vi "Process.vi"(8 "error in":errorcluster, 11 "Inst UI.Magneto":refnum<class "Inst UI.Magneto.lvclass">) -> (0 "error out":errorcluster, 3 "Inst UI.Magneto out":refnum<class "Inst UI.Magneto.lvclass">)   [LabVIEW 2019, in "Inst UI.Magneto.lvclass"]
doc: "---------------------------------------------------------------\nJKI State Machine Objects™\nhttp://jki.net/state-machine-objects/\nCopyright (C) 2005-2015, JKI <info@jki.net>\nALL RIGHTS RESERVEDJKI State Machine Objects (SMO) 1.0.0.5\nJKI - JKI\nCopyright (c) 2016, JKI"
uses:
  Inst UI.Magneto.lvclass
  C:/Program Files (x86)/National Instruments/LabVIEW 2019/vi.lib/JKI/JKI SMO/SMO/SMO.lvclass
  C:/Program Files (x86)/National Instruments/LabVIEW 2019/user.lib/LevyLab/Instrument Framework/SMOs/Instrument UI/Instrument UI.lvclass
  C:/Program Files (x86)/National Instruments/LabVIEW 2019/vi.lib/JKI/JKI SMO/SMO.UI/SMO.UI.lvclass
  Inst.Magneto/Typedefs/Inst.Magneto.Commands--Enum.ctl
  Inst.Magneto/Typedefs/Inst.Magneto.getAll--Cluster.ctl
  Inst.Magneto/Inst.Magneto.lvclass
  C:/Program Files (x86)/National Instruments/LabVIEW 2019/user.lib/LevyLab/Instrument Framework/SMOs/Instrument/Instrument.lvclass
  Inst UI.Magneto.UI--Cluster.ctl
  Inst.Magneto/Typedefs/Inst.Magneto.Configuration--Cluster.ctl
  <userlib>/LevyLab/Instrument Framework/SMOs/Configuration/Configuration.lvclass
  <userlib>/LevyLab/Instrument Framework/SMOs/RemoteControl/Typedefs/Message--Cluster.ctl
  <userlib>/LevyLab/Instrument Framework/SMOs/Instrument UI/Instrument UI.lvclass/Instrument UI.ctl
  Inst.Magneto/Inst.Magneto.lvclass/Inst.Magneto.ctl
  <vilib>/JKI/JKI SMO/SMO/SMO.lvclass/SMO.ctl
  <userlib>/LevyLab/Instrument Framework/SMOs/Configuration/Configuration.lvclass/Configuration.ctl
  <userlib>/LevyLab/Instrument Framework/SMOs/Instrument/Instrument.lvclass/Instrument.ctl
  <userlib>/LevyLab/Instrument Framework/SMOs/Instrument/Typedefs/Client Type--Enum.ctl
  36130e5c-4340-4b59-a0e3-69bc2d3aea66.vi
  09e9697b-516c-49fb-b2dc-692589121b6f.vi
  <vilib>/JKI/JKI SMO/SMO/Private/ReftoDVR--SMO.vi
  09e9697b-516c-49fb-b2dc-692589121b6f.vi/cc30aaa2-4cab-4253-82f5-7584654065fd.vi
  09e9697b-516c-49fb-b2dc-692589121b6f.vi/cc30aaa2-4cab-4253-82f5-7584654065fd.vi/c8a96f78-a4da-4a88-8425-6c4f2c11086a.vi
  <userlib>/LevyLab/Instrument Framework/SMOs/Instrument/API/Send and Receive.vi
  09e9697b-516c-49fb-b2dc-692589121b6f.vi/cc30aaa2-4cab-4253-82f5-7584654065fd.vi/d7be4ad8-201f-4865-b26c-b4f29c6f9adb.vi
  <userlib>/LevyLab/Instrument Framework/SMOs/Instrument/Private/Get Client Type.vi
  09e9697b-516c-49fb-b2dc-692589121b6f.vi/cc30aaa2-4cab-4253-82f5-7584654065fd.vi/c8a96f78-a4da-4a88-8425-6c4f2c11086a.vi/c8de3620-5771-48fc-a831-9cb6daefdad3.vi
  09e9697b-516c-49fb-b2dc-692589121b6f.vi/cc30aaa2-4cab-4253-82f5-7584654065fd.vi/c8a96f78-a4da-4a88-8425-6c4f2c11086a.vi/b35627d4-a654-4984-b331-4a3a395fed01.vi
  09e9697b-516c-49fb-b2dc-692589121b6f.vi/cc30aaa2-4cab-4253-82f5-7584654065fd.vi/d7be4ad8-201f-4865-b26c-b4f29c6f9adb.vi/f494a3ae-3c03-4931-987a-c87ab374a794.vi
  09e9697b-516c-49fb-b2dc-692589121b6f.vi/cc30aaa2-4cab-4253-82f5-7584654065fd.vi/d7be4ad8-201f-4865-b26c-b4f29c6f9adb.vi/582413b9-0fe2-481b-be04-b448e5fee34f.vi
  09e9697b-516c-49fb-b2dc-692589121b6f.vi/cc30aaa2-4cab-4253-82f5-7584654065fd.vi/d7be4ad8-201f-4865-b26c-b4f29c6f9adb.vi/f494a3ae-3c03-4931-987a-c87ab374a794.vi/0ff650d9-b68d-4108-b8b1-733b4d68d29e.vi
  09e9697b-516c-49fb-b2dc-692589121b6f.vi/cc30aaa2-4cab-4253-82f5-7584654065fd.vi/d7be4ad8-201f-4865-b26c-b4f29c6f9adb.vi/f494a3ae-3c03-4931-987a-c87ab374a794.vi/2f422144-46f9-473a-bbc2-4310a8f125b6.vi
  <vilib>/JDP Science/JSONtext/JSON text to Variant.vi
  <userlib>/LevyLab/Instrument Framework/SMOs/Instrument/Private/Get RC Connection Status.vi
  <userlib>/LevyLab/Instrument Framework/SMOs/RemoteControl/API/Send and Receive.vi
  <vilib>/Utility/Data Type/Get Type Information.vi
  <vilib>/JDP Science/JSONtext/Variant to JSON Text.vi
  <vilib>/National Instruments/GUID Generator/Guid Generator.vi
  <userlib>/LevyLab/Instrument Framework/SMOs/Instrument/Private/Instrument.MessageFromProcess.EventStructure.vi
  <userlib>/LevyLab/Instrument Framework/SMOs/Instrument/Instrument.lvclass
  <vilib>/JDP Science/JSONtext/LVClass Serializer/JSONtext LVClass Serializer.lvclass
  <userlib>/LevyLab/Instrument Framework/SMOs/Instrument UI/Instrument UI.lvclass
  <vilib>/JKI/JKI SMO/SMO/SMO.lvclass
  <vilib>/JKI/JKI SMO/SMO.UI/SMO.UI.lvclass
  <userlib>/LevyLab/Instrument Framework/SMOs/RemoteControl/RemoteControl.lvclass
panel:
  out "error out 2":errorcluster
  out "output array":dbl[][](array[numeric])
  out "B-field Values (sensor, x, y, z) uT":cluster{dbl[], dbl[], dbl[], dbl[]}
  out "coerced(x)":u32
  out "Sensor 0 B_y":dbl(graph)
  out "Sensor 0 B_x":dbl(graph)
  in  "STOP":bool
  # "SMO UI Template"
  # "For instructions on how to use the JKI State Machine Objects, examples and video tutorials, visit:\nhttp://jki.net/state-machine-objects/\n\nJKI State Machine Objects™\nhttp://jki.net/state-machine-objects/\nCopyright (C) 2005-2015, JKI <info@jki.net>\nALL RIGHTS RESERVED"
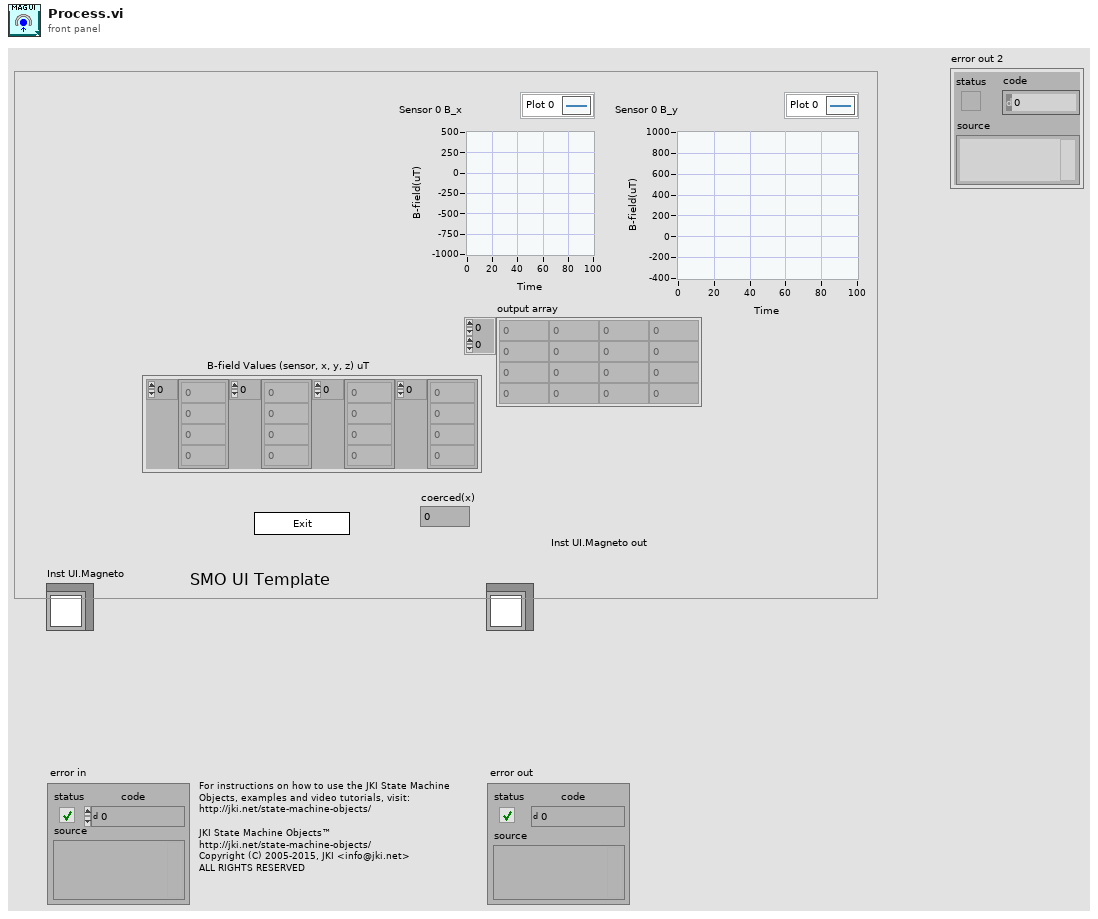
[diagram p1: front panel]
types:
  T1 = typedef "Inst.Magneto.lvclass/Inst.Magneto.Commands--Enum.ctl" = enum16{"GetRead", "Read", "Clear Values"}
  T2 = enum32{"invalid app kind", "Development System", "Run Time System", "Student Edition", "Embedded LabVIEW", "Evaluation", "Custom"}
  T3 = typedef "Inst.Magneto.lvclass/Inst.Magneto.getAll--Cluster.ctl" = cluster{"AllString":string}
  T4 = cluster{"Sensor":i32, "x":dbl, "y":dbl, "z":dbl}[]
  T5 = enum32{"Invalid", "Standard", "Closed", "Hidden", "Minimized", "Maximized"}
  T6 = typedef "Instrument.lvclass/Client Type--Enum.ctl" = enum16{"Remote", "Local"}
  T7 = typedef "Inst.Magneto.lvclass/Inst.Magneto.Configuration--Cluster.ctl" = cluster{"Server URL":string}
  T8 = typedef "Inst UI.Magneto.lvclass/Inst UI.Magneto.UI--Cluster.ctl" = cluster{"Parameter":dbl, "\nURL":string}
  T9 = typedef "RemoteControl.lvclass/Message--Cluster.ctl" = cluster{"Command":string, "Data":variant, "ID":string}
  T10 = cluster{"Core":cluster{"Current VI Reference":refnum<vi>, "Close Panel on Exit?":bool, "Last Error":cluster{"error":errorcluster, "previous state":string, "remaining states":string}, "Shutdown?":bool}, "Instrument UI":refnum<class "Inst UI.Magneto.lvclass">, "Instrument":refnum<class "Inst.Magneto.lvclass">, "Configuration":refnum<class "Configuration.lvclass">, "Config Cluster":T7, "getAll":T3, "UI Cluster":T8, "Message":T9}
  T11 = cluster{"Current VI Reference":refnum<vi>, "Close Panel on Exit?":bool, "Last Error":cluster{"error":errorcluster, "previous state":string, "remaining states":string}, "Shutdown?":bool}
  T12 = typedef "SMO.lvclass/Protected Events.ctl" = cluster{"StopProcesses":refnum<user-event>, "AbortProcesses":refnum<user-event>, "Config Changed":refnum<user-event>, "Dependency":refnum<user-event>}
  T13 = typedef "Instrument.lvclass/PublicEvents--Cluster.ctl" = cluster{"MessageFromProcess":refnum<user-event>}
  T14 = typedef "Inst.Magneto.lvclass/PublicEvents--Cluster.ctl" = cluster{"MessageFromProcess":refnum<user-event>}
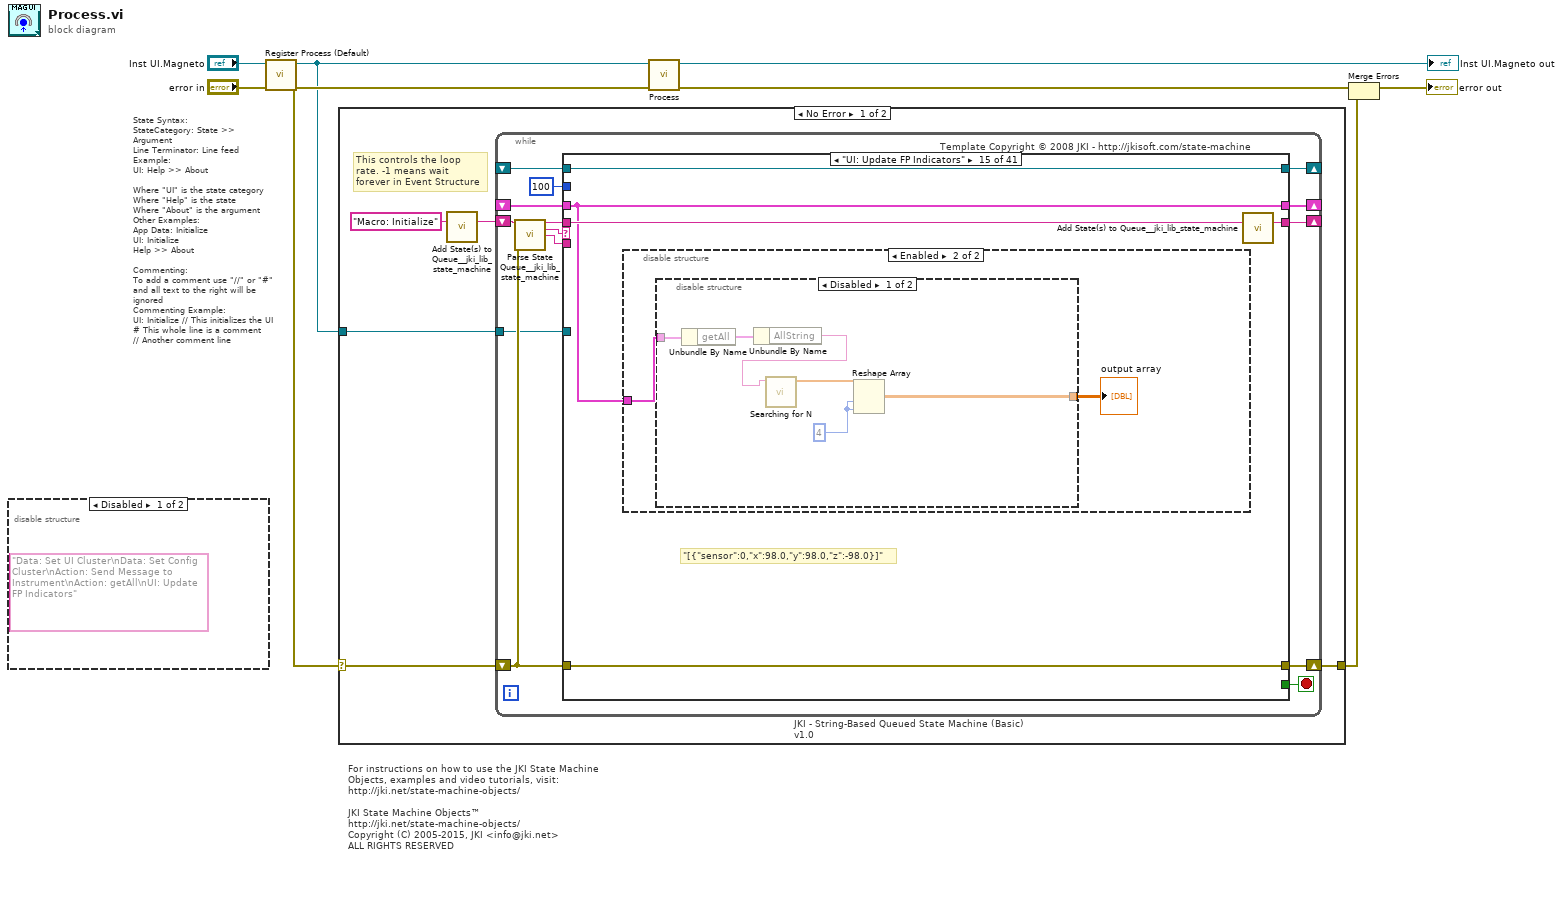
[diagram p0: block diagram]
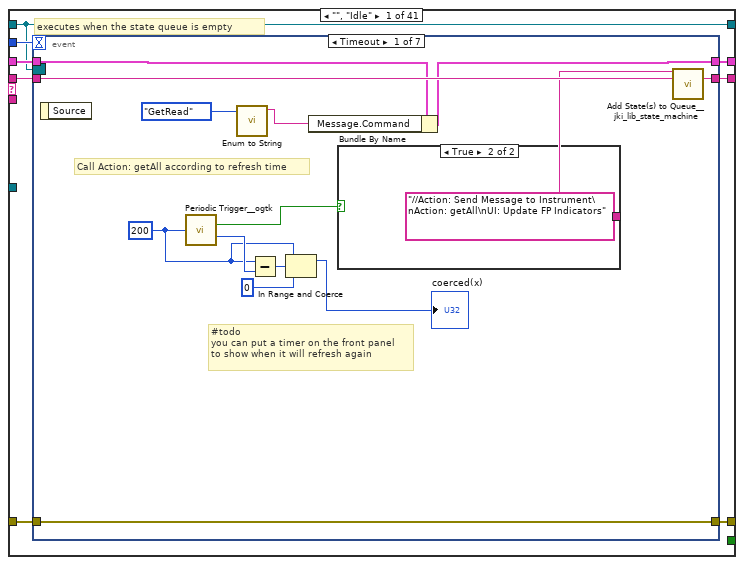
[diagram p3: hidden frame]
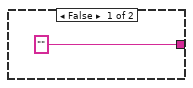
[diagram p4: hidden frame]
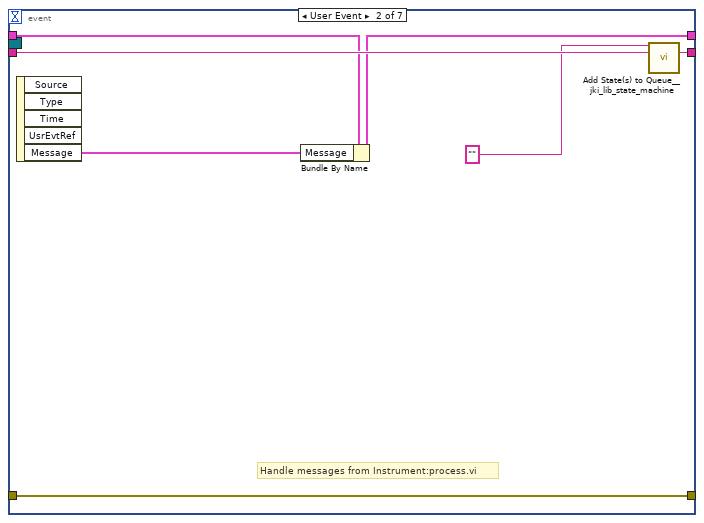
[diagram p5: hidden frame]
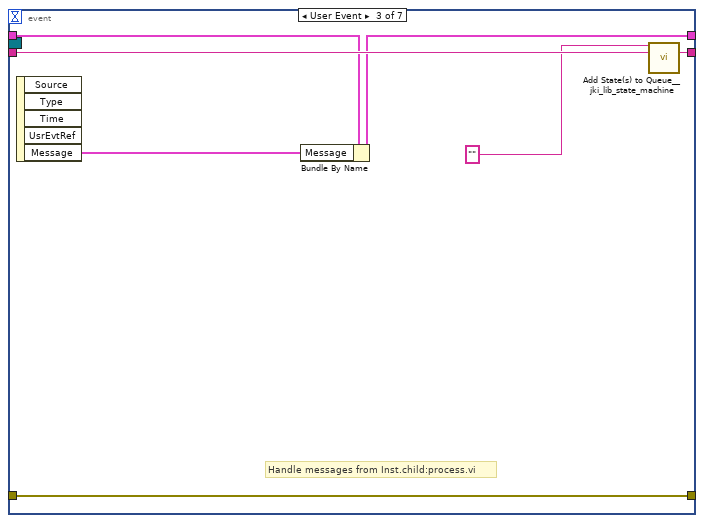
[diagram p6: hidden frame]
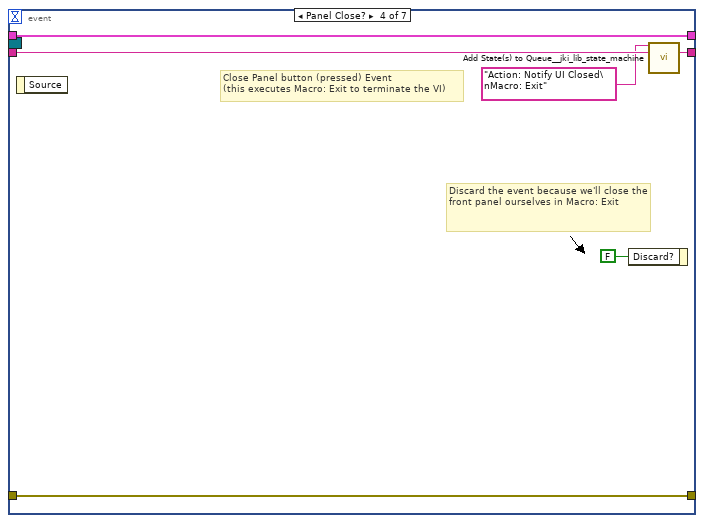
[diagram p7: hidden frame]
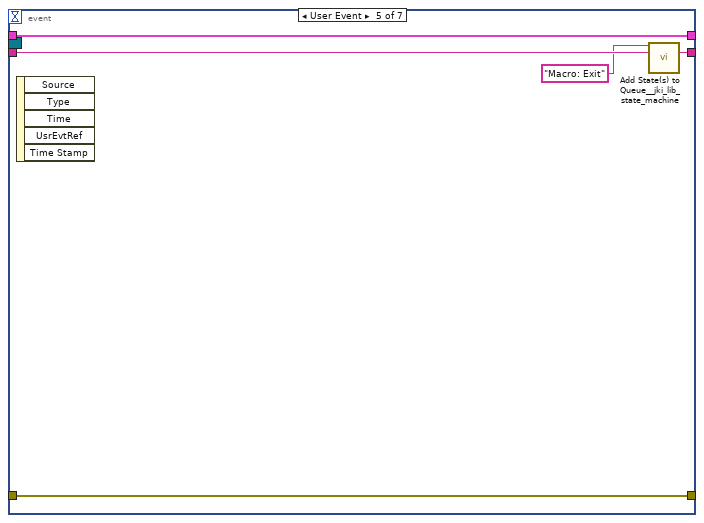
[diagram p8: hidden frame]
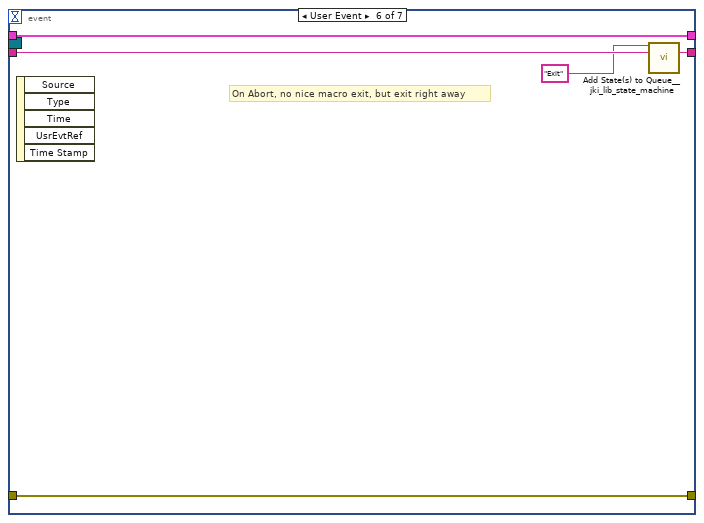
[diagram p9: hidden frame]
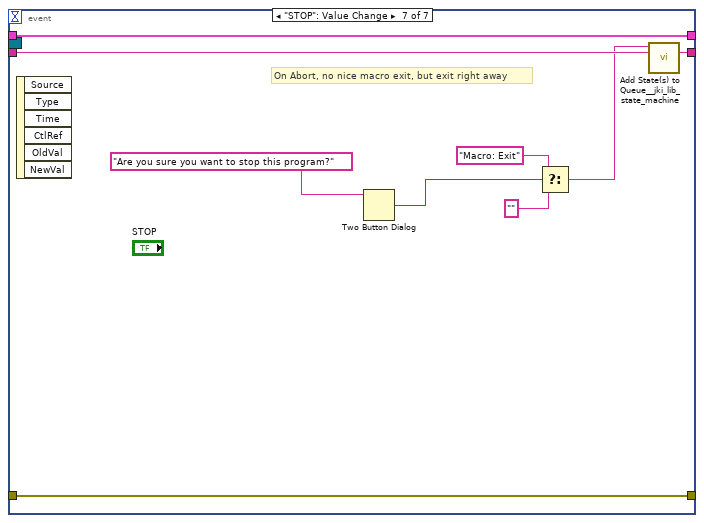
[diagram p10: hidden frame]
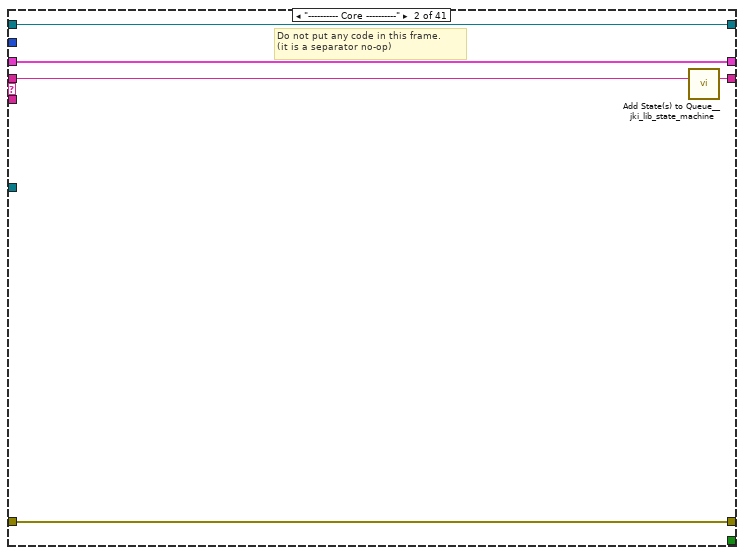
[diagram p11: hidden frame]
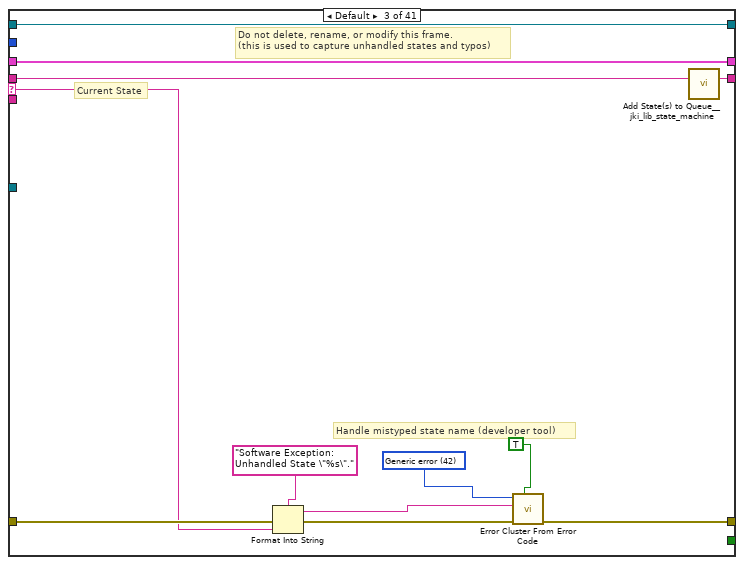
[diagram p12: hidden frame]
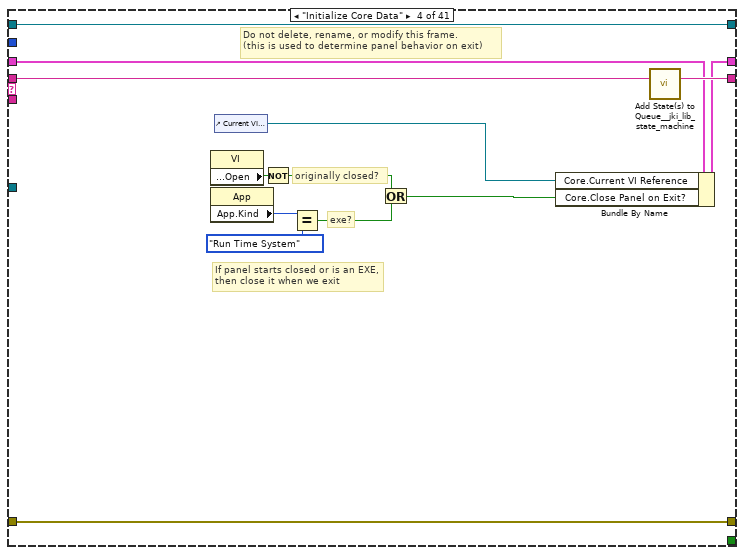
[diagram p13: hidden frame]
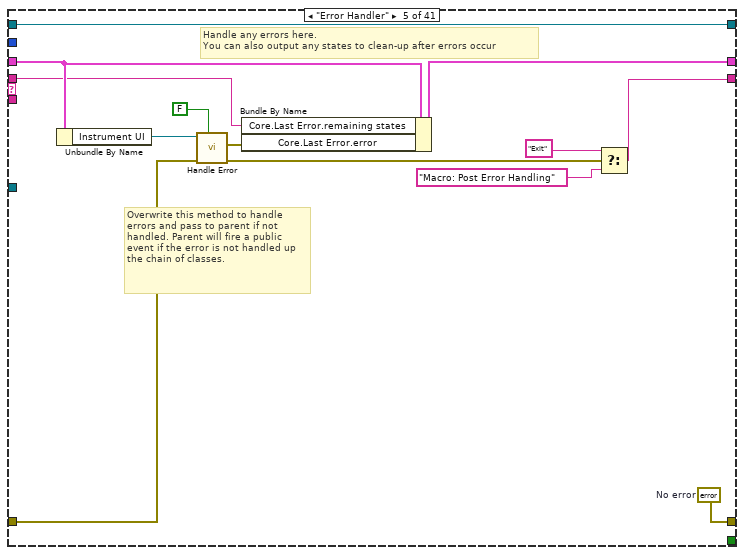
[diagram p14: hidden frame]
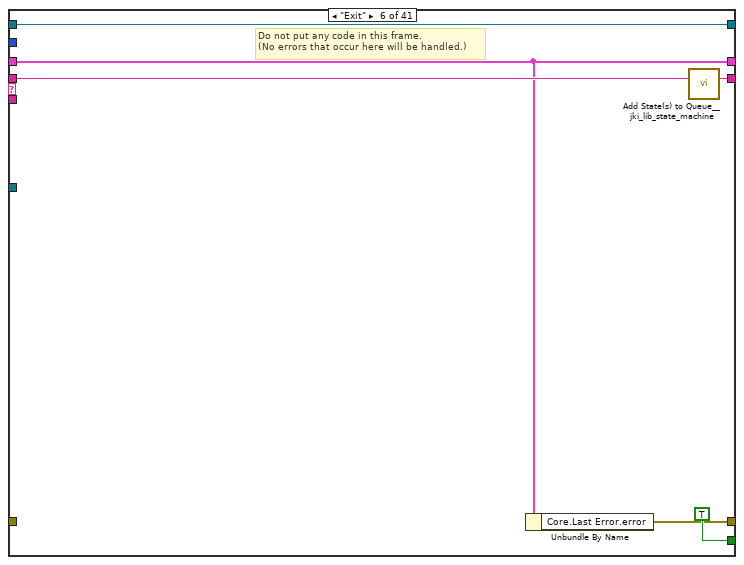
[diagram p15: hidden frame]
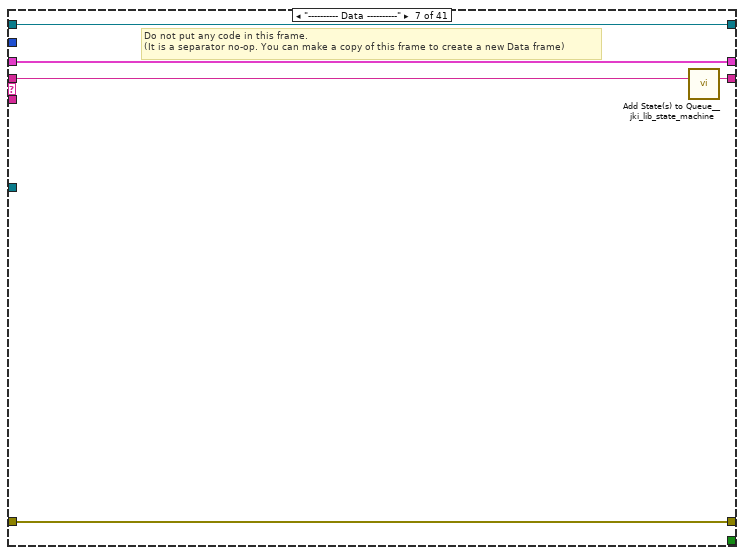
[diagram p16: hidden frame]
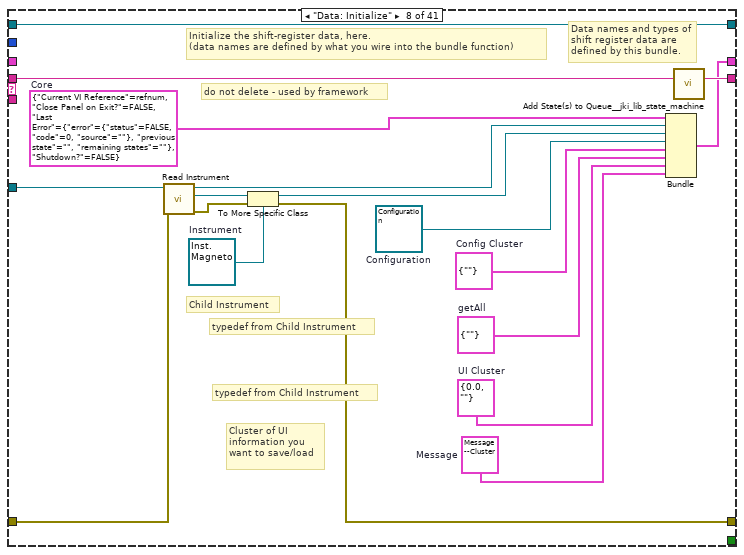
[diagram p17: hidden frame]
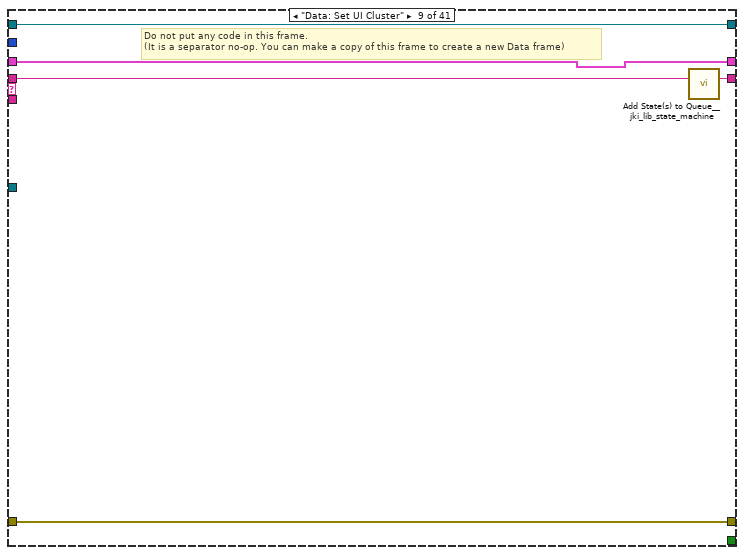
[diagram p18: hidden frame]
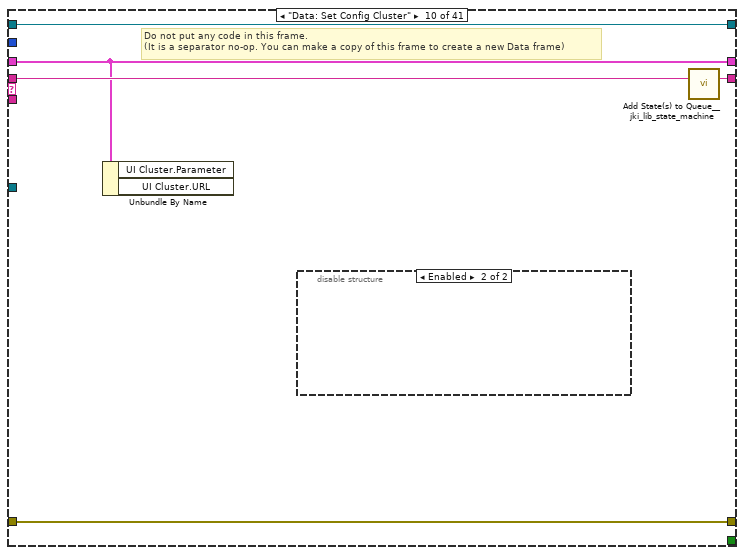
[diagram p19: hidden frame]
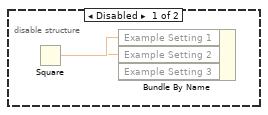
[diagram p20: hidden frame]
diagram:
  # "State Syntax:\nStateCategory: State >> Argument\nLine Terminator: Line feed\nExample:\nUI: Help >> About\n\nWhere \"UI\" is the state category\nWhere \"Help\" is the state\nWhere \"About\" is the argument\nOther Examples:\nApp Data: Initialize\nUI: Initialize\nHelp >> About\n\nCommenting:\nTo add a comment use \"//\" or \"#\" and all text to the right will be ignored\nCommenting Example:\nUI: Initialize // This initializes the UI\n# This whole line is a comment\n// Another comment line"
  # "For instructions on how to use the JKI State Machine Objects, examples and video tutorials, visit:\nhttp://jki.net/state-machine-objects/\n\nJKI State Machine Objects™\nhttp://jki.net/state-machine-objects/\nCopyright (C) 2005-2015, JKI <info@jki.net>\nALL RIGHTS RESERVED"
  n1 = disable-structure shown="Disabled" {
    frame Disabled {
      w9 = "Data: Set UI Cluster\nData: Set Config Cluster\nAction: Send Message to Instrument\nAction: getAll\nUI: Update FP Indicators" ("State(s) in Front (\"\")")
    }
    frame Enabled {
    }
  }
  n2 = call <vilib>:"Register Process (Default).vi"("error in (no error)"="error in", "SMO"="Inst UI.Magneto") -> ("error out"=w5:errorcluster, "SelfRef"=w4:refnum<class "Inst UI.Magneto.lvclass">)  [unwired: 8 in]
  n3 = case shown="No Error" w5 {
    selector: w5 -> [w11 w513]
    tunnel: w4 -> [w12 _]
    tunnel: [w10 w513] -> w1
    frame No Error {
      # "This controls the loop rate. -1 means wait forever in Event Structure"
      n4 = call <vilib>:"Add State(s) to Queue__jki_lib_state_machine.vi"("State(s) in (\"\")"="Macro: Initialize") -> ("States Out"=w14:string)  [unwired: 14 in]
      n5 = while "JKI - String-Based Queued State Machine (Basic) v1.0" {
        shift-right: [w21] -> _
        shift-left: _ -> [w20]
        shift-right: [w24] -> w10
        shift-left: w11 -> [w18]
        shift-right: [w23] -> _
        shift-left: w14 -> [w25]
        tunnel: w12 -> [w17]
        shift-right: [w16] -> _
        shift-left: _ -> [w15]
        stop <- w22 stop-if-true
        # "Template Copyright © 2008 JKI - http://jkisoft.com/state-machine"
        n6 = call <vilib>:"Parse State Queue__jki_lib_state_machine.vi"("State Queue"=w25, "Error In (no error)"=w18) -> ("Remaining States"=w27:string, "Current State"=w28:string, "Arguments"=w26:string)  [unwired: 11 in]
        n7 = case shown="\"UI: Update FP Indicators\"" w28 {
          selector: w28 -> [_ _ w98 _ _ _ _ _ _ _ _ _ _ _ _ _ _ _ _ _ _ _ _ _ _ _ _ _ _ _ _ _ _ _ _ _ _ _ _ _ _]
          tunnel: w27 -> [w36 w96 w102 w121 w125 w140 w145 w163 w168 w173 w183 w188 w195 w200 w205 w241 w257 w289 w298 w310 w320 w326 w341 w346 w357 w364 w369 w385 w391 w396 w411 w419 w431 w438 w445 w457 w470 w480 w491 w502 w512]
          tunnel: w26 -> [_ _ _ _ _ _ _ _ _ _ _ _ _ _ _ w235 w251 _ _ _ _ _ _ _ _ _ _ _ _ _ _ _ _ _ _ _ _ _ _ _ _]
          tunnel: w20 -> [w34 w93 w100 w112 w128 w136 w142 _ w164 w169 w177 w185 w193 w196 w201 w239 w253 w286 w294 w300 w317 w323 w328 w343 w354 w359 w366 w383 w389 w393 w404 w416 w422 w433 w439 w449 w464 w472 w486 w497 w507]
          tunnel: [w33 w94 w104 w118 w130 w135 w143 w150 w166 w171 w179 w186 w190 w198 w202 w236 w254 w287 w296 w308 w318 w324 w339 w344 w348 w360 w367 w380 w386 w394 w397 w414 w423 w435 w440 w454 w467 w477 w482 w493 w503] -> w24
          tunnel: w18 -> [w32 w94 w103 w118 w124 _ w143 w147 w166 w171 w180 w186 w191 w198 w202 w237 w255 w287 w296 w308 w318 w324 w339 w344 w349 w361 w367 w370 w387 w394 w406 w412 w424 w435 w441 w450 w459 w473 w483 w494 w504]
          tunnel: [w35 w95 w101 w120 w122 w139 w144 w162 w167 w172 w182 w187 w194 w199 w204 w240 w256 w288 w297 w309 w319 w325 w340 w345 w356 w363 w368 w384 w390 w395 w410 w418 w430 w437 w444 w456 w469 w479 w490 w501 w511] -> w23
          tunnel: [_ _ _ _ _ TRUE _ _ _ _ _ _ _ _ _ _ _ _ _ _ _ _ _ _ _ _ _ _ _ _ _ _ _ _ _ _ _ _ _ _ _] -> w22
          tunnel: [w31 w93 w100 w119 w127 w136 w142 w161 w164 w169 w177 w185 w193 w196 w201 w239 w253 w286 w294 w301 w317 w323 w328 w343 w354 w359 w366 w383 w389 w393 w408 w416 w420 w432 w439 w451 w465 w474 w487 w498 w508] -> w21
          tunnel: 100 ("Timeout") -> [w30 _ _ _ _ _ _ _ _ _ _ _ _ _ _ _ _ _ _ _ _ _ _ _ _ _ _ _ _ _ _ _ _ _ _ _ _ _ _ _ _]
          tunnel: w17 -> [_ _ _ _ _ _ _ w148 _ _ _ _ _ _ _ _ _ _ _ _ _ _ _ _ _ _ _ _ _ _ _ _ _ _ _ _ _ _ _ _ _]
          tunnel: [w29 w92 w97 w109 w134 w137 w141 w160 w165 w170 w178 w184 w192 w197 w203 w238 w250 w285 w295 w307 w316 w322 w333 w342 w355 w362 w365 w382 w388 w392 w409 w417 w429 w436 w443 w455 w468 w478 w489 w500 w510] -> w16
          tunnel: w15 -> [w29 w92 w97 w109 w134 w137 w141 w160 w165 w170 w178 w184 w192 w197 w203 w238 w250 w285 w295 w307 w316 w322 w333 w342 w355 w362 w365 _ w388 w392 w409 w417 w429 w436 w443 w455 w468 w478 w489 w500 w510]
          frame "", "Idle" {
            # "executes when the state queue is empty"
            n8 = event shown="[0] Timeout" {
              selector: w29 -> [_ _ _ _ _ _ _]
              dyn-events: _ -> [_ _ _ _ _ _ _]
              timeout: w30 -> [_ _ _ _ _ _ _]
              tunnel: w36 -> [w50 w59 w66 w72 w77 w82 w91]
              tunnel: [w49 w58 w65 w71 w76 w81 w90] -> w35
              tunnel: w34 -> [w39 w56 w63 w68 w74 w79 w88]
              tunnel: [w48 w57 w64 w67 w75 w80 w89] -> w33
              tunnel: w32 -> [w48 w57 w64 w67 w75 w80 w89]
              tunnel: [w40 w55 w62 w68 w74 w79 w88] -> w31
              event Timeout {
                w43 = u32 200 ("time (ms)")
                # "#todo\nyou can put a timer on the front panel\nto show when it will refresh again"
                # "Call Action: getAll according to refresh time"
                n9 = event-data() -> ()  [unwired: 1 in, 1 out]
                n10 = call <userlib>:"Periodic Trigger__ogtk.vi"("time (ms)"=w43) -> ("Triggered"=w47:bool, "timer value"=w46:u32)  [unwired: 12 in, 1 out]
                n11 = call <userlib>:"Enum to String.vi"("Command"=Inst.Magneto.Commands--Enum."GetRead" ("Commands")) -> ("Command"=w37:string)  [unwired: 9 in, 1 out]
                n12 = Subtract(x=w43, y=w46) -> (x-y=w45:u32)
                n13 = In Range and Coerce(upper limit=w43, x=w45, lower limit=u32 0) -> (coerced(x)=→"coerced(x)":u32)  [unwired: 1 out]
                n14 = Bundle By Name(cluster=w39, "Message.Command"=w37) -> (w40:T10)
                n15 = case shown="True" w47 {
                  tunnel: ["" ("State(s) in Front (\"\")") "//Action: Send Message to Instrument\nAction: getAll\nUI: Update FP Indicators" ("State(s) in Front (\"\")")] -> w41
                  frame False {
                  }
                  frame True {
                  }
                }
                n16 = call <vilib>:"Add State(s) to Queue__jki_lib_state_machine.vi"("State(s) in Front (\"\")"=w41, "State(s) in (\"\")"=w50) -> ("States Out"=w49:string)  [unwired: 13 in]
              }
              event User Event {
                # "Handle messages from Instrument:process.vi"
                n17 = event-data() -> ("Message"=w53:T9)  [unwired: 1 in, 4 out]
                n18 = Bundle By Name(cluster=w56, "Message"=w53) -> (w55:T10)
                n19 = call <vilib>:"Add State(s) to Queue__jki_lib_state_machine.vi"("State(s) in Front (\"\")"="" ("State(s) in Front (\"\")"), "State(s) in (\"\")"=w59) -> ("States Out"=w58:string)  [unwired: 13 in]
              }
              event User Event {
                # "Handle messages from Inst.child:process.vi"
                n20 = event-data() -> ("Message"=w60:T9)  [unwired: 1 in, 4 out]
                n21 = Bundle By Name(cluster=w63, "Message"=w60) -> (w62:T10)
                n22 = call <vilib>:"Add State(s) to Queue__jki_lib_state_machine.vi"("State(s) in Front (\"\")"="" ("State(s) in Front (\"\")"), "State(s) in (\"\")"=w66) -> ("States Out"=w65:string)  [unwired: 13 in]
              }
              event Panel Close? {
                # "Discard the event because we'll close the front panel ourselves in Macro: Exit"
                # "Close Panel button (pressed) Event\n(this executes Macro: Exit to terminate the VI)"
                n23 = event-data() -> ()  [unwired: 1 in, 1 out]
                n24 = event-data("Discard?"=FALSE) -> ()  [unwired: 1 in, 1 out]
                n25 = call <vilib>:"Add State(s) to Queue__jki_lib_state_machine.vi"("State(s) in Front (\"\")"="Action: Notify UI Closed\nMacro: Exit", "State(s) in (\"\")"=w72) -> ("States Out"=w71:string)  [unwired: 13 in]
              }
              event User Event {
                n26 = event-data() -> ()  [unwired: 1 in, 5 out]
                n27 = call <vilib>:"Add State(s) to Queue__jki_lib_state_machine.vi"("State(s) in Front (\"\")"="Macro: Exit", "State(s) in (\"\")"=w77) -> ("States Out"=w76:string)  [unwired: 13 in]
              }
              event User Event {
                # "On Abort, no nice macro exit, but exit right away"
                n28 = event-data() -> ()  [unwired: 1 in, 5 out]
                n29 = call <vilib>:"Add State(s) to Queue__jki_lib_state_machine.vi"("State(s) in Front (\"\")"="Exit", "State(s) in (\"\")"=w82) -> ("States Out"=w81:string)  [unwired: 13 in]
              }
              event "STOP": Value Change {
                # "On Abort, no nice macro exit, but exit right away"
                n30 = event-data() -> ()  [unwired: 1 in, 6 out]
                n31 = Two Button Dialog(message="Are you sure you want to stop this program?") -> (T button?=w87:bool)  [unwired: 2 in]
                n32 = Select(t="Macro: Exit", s=w87, f="") -> (s? t:f=w83:string)
                n33 = call <vilib>:"Add State(s) to Queue__jki_lib_state_machine.vi"("State(s) in Front (\"\")"=w83, "State(s) in (\"\")"=w91) -> ("States Out"=w90:string)  [unwired: 13 in]
              }
            }
          }
          frame "---------- Core ----------" {
            # "Do not put any code in this frame.\n(it is a separator no-op)"
            n34 = call <vilib>:"Add State(s) to Queue__jki_lib_state_machine.vi"("State(s) in (\"\")"=w96) -> ("States Out"=w95:string)  [unwired: 14 in]
          }
          frame Default {
            w107 = 42 items=["No error", "Argument error", "Memory is full", "Out of zone", "End of file", "File already open", "Generic file I/O error", "File not found", "File permission error", "Disk is full", "Duplicate path", "Too many files open", "System feature not enabled", "Resource file not found", "Cannot add resource", "Resource not found", "Image not found", "Image memory error", "Pen does not exist", "Config type invalid", "Config token not found", "Config parse error", "Config memory error", "Bad external code format", "Bad external code offset", "External code not present", "Null window", "Destroy window error", "Null menu", "Print aborted", "Bad print record", "Print driver error", "Windows error during printing", "Memory error during printing", "Print dialog error", "Generic print error", "Invalid device refnum", "Device not found", "Device parameter error", "Device unit error", "Cannot open device", "Device call aborted", "Generic error", "Cancelled by user", "Object ID too low", "Object ID too high", "Object not in heap", "Unknown heap", "Unknown object (invalid DefProc)", "Unknown object (DefProc not in table)", "Message out of range", "Invalid (null) method", "Unknown message", "Manager call not supported", "Bad address", "Network operation in progress", "Network operation timed out", "Connection is busy", "Network attribute not supported", "Network error", "Address in use", "System out of memory", "Connection aborted", "Connection refused", "Not connected", "Already connected", "Connection closed", "Initialization error (interapplication manager)", "Bad occurrence", "Wait on unbound occurrence handler", "Occurrence queue overflow", "Datalog type conflict", "Unused", "Unrecognized type (interapplication manager)", "Memory corrupt", "Failed to make temporary DLL", "Old CIN version", "Drag socket not found", "Failed to load drop-object", "Failed to register OLE object", "Failed to release OLE object", "Format specifier type mismatch", "Unknown format specifier", "Too few format specifiers", "Too many format specifiers", "Scan failed", "Newer CIN version", "Error converting to variant", "Runtime menu error", "Password tampered", "Variant attribute not found", "Incompatible variant data type", "Event data is not available", "Event Store is not present", "Occurrence is not found", "Event Queue is not created", "Event info is not available", "Refnum passed is NULL", "Error retrieving Class GUID", "Error retrieving CoClass GUID", "Error retrieving TypeLib GUID.", "Bad built application magic bytes.", "Specific driver is different from the specific driver associated with the Logical Name.", "There is no session opened to the class driver.", "Max Error", "MAX - Error with config objects", "MAX - Error loading configuration", "MAX - Group not supported"]
            # "Current State"
            # "Do not delete, rename, or modify this frame.\n(this is used to capture unhandled states and typos)"
            # "Handle mistyped state name (developer tool)"
            n35 = Format Into String(format string="Software Exception: Unhandled State \"%s\"." ("message"), error in=w103, w98) -> (resulting string=w106:string, error out=w105:errorcluster)  [unwired: 1 in]
            n36 = call <vilib>:"Error Cluster From Error Code.vi"("show call chain? (False)"=TRUE, "error in (no error)"=w105, "error message (\"\")"=w106, "error code (0)"=w107) -> ("error out"=w104:errorcluster)  [unwired: 5 in]
            n37 = call <vilib>:"Add State(s) to Queue__jki_lib_state_machine.vi"("State(s) in (\"\")"=w102) -> ("States Out"=w101:string)  [unwired: 14 in]
          }
          frame "Initialize Core Data" {
            # "Do not delete, rename, or modify this frame.\n(this is used to determine panel behavior on exit)"
            # "originally closed?"
            # "exe?"
            # "If panel starts closed or is an EXE, then close it when we exit"
            n38 = property class="VI"() -> ("Front Panel.Open"=w117:bool)  [unwired: 2 in, 2 out]
            n39 = property class="App"() -> ("App.Kind"=w116:T2)  [unwired: 2 in, 2 out]
            n40 = control-ref of="Current VI Reference"() -> (w110:refnum<vi>)
            n41 = Not(x=w117) -> (.not. x?=w114:bool)
            n42 = Equal?(x=w116, y=T2."Run Time System" ("Application:Kind")) -> (x = y?=w113:bool)
            n43 = Or(x=w114, y=w113) -> (x .or. y?=w111:bool)
            n44 = Bundle By Name(cluster=w112, "Core.Current VI Reference"=w110, "Core.Close Panel on Exit?"=w111) -> (w119:T10)
            n45 = call <vilib>:"Add State(s) to Queue__jki_lib_state_machine.vi"("State(s) in (\"\")"=w121) -> ("States Out"=w120:string)  [unwired: 14 in]
          }
          frame "Error Handler" {
            w130 = errorcluster {"status"=FALSE, "code"=0, "source"=""}  # No error
            # "Overwrite this method to handle errors and pass to parent if not handled. Parent will fire a public event if the error is not handled up the chain of classes."
            # "Handle any errors here.\nYou can also output any states to clean-up after errors occur"
            n46 = Unbundle By Name(w128) -> ("Instrument UI"=w133:refnum<class "Inst UI.Magneto.lvclass">)
            n47 = call-dynamic "Handle Error.vi"("Stop on Unhandled Error (T)"=FALSE, "error in"=w124, "SMO"=w133) -> ("handling error"=w131:errorcluster, "Unhandled error"=w129:errorcluster)  [unwired: 6 in, 1 out]
            n48 = Bundle By Name(cluster=w128, "Core.Last Error.remaining states"=w125, "Core.Last Error.error"=w129) -> (w127:T10)
            n49 = Select(t="Exit", s=w131, f="Macro: Post Error Handling") -> (s? t:f=w122:string)
          }
          frame "Exit" {
            # "Do not put any code in this frame.\n(No errors that occur here will be handled.)"
            n50 = Unbundle By Name(w136) -> ("Core.Last Error.error"=w135:errorcluster)
            n51 = call <vilib>:"Add State(s) to Queue__jki_lib_state_machine.vi"("State(s) in (\"\")"=w140) -> ("States Out"=w139:string)  [unwired: 14 in]
          }
          frame "---------- Data ----------" {
            # "Do not put any code in this frame.\n(It is a separator no-op. You can make a copy of this frame to create a new Data frame)"
            n52 = call <vilib>:"Add State(s) to Queue__jki_lib_state_machine.vi"("State(s) in (\"\")"=w145) -> ("States Out"=w144:string)  [unwired: 14 in]
          }
          frame "Data: Initialize" {
            w146 = T9 {"Command"="", "Data"=variant, "ID"=""}  # Message
            w149 = refnum<class "Configuration.lvclass"> refnum  # Configuration
            w152 = T7 {"Server URL"=""}  # Config Cluster
            w154 = T8 {"Parameter"=0.0, "\nURL"=""}  # UI Cluster
            w156 = refnum<class "Inst.Magneto.lvclass"> refnum  # Instrument
            w158 = T3 {"AllString"=""}  # getAll
            w159 = T11 {"Current VI Reference"=refnum, "Close Panel on Exit?"=FALSE, "Last Error"={"error"={"status"=FALSE, "code"=0, "source"=""}, "previous state"="", "remaining states"=""}, "Shutdown?"=FALSE}  # Core
            # "typedef from Child Instrument"
            # "Cluster of UI\ninformation you\nwant to save/load"
            # "Child Instrument"
            # "typedef from Child Instrument"
            # "do not delete - used by framework"
            # "Data names and types of shift register data are defined by this bundle."
            # "Initialize the shift-register data, here.\n(data names are defined by what you wire into the bundle function)"
            n53 = call <userlib>:"Read Instrument.vi"("error in (no error)"=w147, "Instrument UI in"=w148) -> ("error out"=w153:errorcluster, "Instrument"=w155:refnum<class "Instrument.lvclass">, "Instrument UI"=w157:refnum<class "Inst UI.Magneto.lvclass">)  [unwired: 7 in]
            n54 = To More Specific Class(target class=w156, reference=w155, error in=w153) -> (specific class reference=w151:refnum<class "Inst.Magneto.lvclass">, error out=w150:errorcluster)
            n55 = Bundle("Core"=w159, "Instrument UI"=w157, "Instrument"=w151, "Configuration"=w149, "Config Cluster"=w152, "getAll"=w158, "UI Cluster"=w154, "Message"=w146) -> (w161:T10)  [unwired: 1 in]
            n56 = call <vilib>:"Add State(s) to Queue__jki_lib_state_machine.vi"("State(s) in (\"\")"=w163) -> ("States Out"=w162:string)  [unwired: 14 in]
          }
          frame "Data: Set UI Cluster" {
            # "Do not put any code in this frame.\n(It is a separator no-op. You can make a copy of this frame to create a new Data frame)"
            n57 = call <vilib>:"Add State(s) to Queue__jki_lib_state_machine.vi"("State(s) in (\"\")"=w168) -> ("States Out"=w167:string)  [unwired: 14 in]
          }
          frame "Data: Set Config Cluster" {
            # "Do not put any code in this frame.\n(It is a separator no-op. You can make a copy of this frame to create a new Data frame)"
            n58 = Unbundle By Name(w169) -> ()  [unwired: 2 out]
            n59 = disable-structure shown="Enabled" {
              frame Disabled {
                n60 = Square(x=w175) -> (x^2=w174:dbl)
                n61 = Bundle By Name("Example Setting 2"=w174) -> ("Example Setting 1"=w175:dbl, "Example Setting 3"=w176:string)  [unwired: 1 in, 1 out]
              }
              frame Enabled {
              }
            }
            n62 = call <vilib>:"Add State(s) to Queue__jki_lib_state_machine.vi"("State(s) in (\"\")"=w173) -> ("States Out"=w172:string)  [unwired: 14 in]
          }
          frame "Data: Cleanup" {
            # "Cleanup any data and references, here.\n(this is called automatically, by the Macro: Exit)"
            n63 = Unbundle By Name(w177) -> ("Core.Current VI Reference"=w181:refnum<vi>)
            n64 = Close Reference(reference=w181, error in (no error)=w180) -> (error out=w179:errorcluster)
            n65 = call <vilib>:"Add State(s) to Queue__jki_lib_state_machine.vi"("State(s) in (\"\")"=w183) -> ("States Out"=w182:string)  [unwired: 14 in]
          }
          frame "---------- UI ----------" {
            # "Do not put any code in this frame.\n(It is a separator no-op. You can make a copy of this frame to create a new UI frame)"
            n66 = call <vilib>:"Add State(s) to Queue__jki_lib_state_machine.vi"("State(s) in (\"\")"=w188) -> ("States Out"=w187:string)  [unwired: 14 in]
          }
          frame "UI: Initialize" {
            # "size window to decoration box on front panel"
            # "Initialize the User Interface, here.\n(this is called automatically, by the Macro: Init)"
            n67 = invoke on="STOP" class="Bool (strict)" method="Reinit To Default"() -> ()  [unwired: 3 in, 3 out]
            n68 = call <userlib>:"Fit VI window to Largest Dec__ogtk.vi"("error in (no error)"=w191, "border spacing (2 px)"=0) -> ("error out"=w190:errorcluster)  [unwired: 4 in, 1 out]
            n69 = call <vilib>:"Add State(s) to Queue__jki_lib_state_machine.vi"("State(s) in (\"\")"=w195) -> ("States Out"=w194:string)  [unwired: 14 in]
          }
          frame "UI: Update FP Controls" {
            # "Do not put any code in this frame.\n(It is a separator no-op. You can make a copy of this frame to create a new UI frame)"
            n70 = call <vilib>:"Add State(s) to Queue__jki_lib_state_machine.vi"("State(s) in (\"\")"=w200) -> ("States Out"=w199:string)  [unwired: 14 in]
          }
          frame "UI: Update FP Indicators" {
            # "\"[{\"sensor\":0,\"x\":98.0,\"y\":98.0,\"z\":-98.0}]\""
            n71 = disable-structure shown="Enabled" {
              disable-tunnel: w201 -> [w216 w218]
              frame Disabled {
                # "do this way to have nicer UI or only display what you want"
                n72 = Unbundle By Name(w216) -> ("Sensor 0"=w206, "Sensor 1"=w209, "Sensor 2"=w208, "Sensor 3"=w207)
                n73 = Bundle By Name(cluster=T3 {"AllString"=""} ("getAll"), "Sensor 0"=w206, "Sensor 1"=w209, "Sensor 2"=w208, "Sensor 3"=w207) -> (→"B-field Values (sensor, x, y, z) uT":T3)
                n74 = Index Array(array=w206, index=1 ("index (row)")) -> (element=→"Sensor 0 B_x")
                n75 = Index Array(array=w206, index=2 ("index (row)")) -> (element=→"Sensor 0 B_y")
              }
              frame Enabled {
                n76 = disable-structure shown="Disabled" {
                  disable-tunnel: w218 -> [w222 w229]
                  disable-tunnel: [w221 w225] -> w217
                  frame Disabled {
                    w223 = 4 ("dimension size")
                    n77 = Unbundle By Name(w222) -> ("getAll"=w220:T3)
                    n78 = Unbundle By Name(w220) -> ("AllString"=w219:string)
                    n79 = call "Searching for N.vi"("body"=w219) -> ("Array"=w224:dbl[])  [unwired: 10 in]
                    n80 = Reshape Array(w224, w223, w223) -> (w221:dbl[][])
                  }
                  frame Enabled {
                    n81 = Unbundle By Name(w229) -> ("getAll.AllString"=w228:string)
                    n82 = call "From JSON Text.vim"("Data Type and Default Value"=T4 [], "JSON"=w228) -> ("Data out"=w226:T4)  [unwired: 8 in, 1 out]
                    n83 = for {
                      tunnel: w226 -> [w234] mode=indexing
                      tunnel: [w230] -> w225 mode=indexing
                      n84 = Unbundle By Name(w234) -> ("x"=w233:dbl, "y"=w232:dbl, "z"=w231:dbl)  [unwired: 1 out]
                      n85 = Build Array(w233, w232, w231) -> (w230:dbl[])
                    }
                  }
                }
                "output array" <- w217
              }
            }
            n86 = call <vilib>:"Add State(s) to Queue__jki_lib_state_machine.vi"("State(s) in (\"\")"=w205) -> ("States Out"=w204:string)  [unwired: 14 in]
          }
          frame "UI: Cursor Set" {
            # "Argument"
            # "Initialize the User Interface, here.\n(this is called automatically, by the Macro: Init)"
            n87 = disable-structure shown="Default" {
              disable-tunnel: w237 -> [w242 w245]
              disable-tunnel: [w242 w244] -> w236
              disable-tunnel: w235 -> [_ w243]
              frame condition #0 {
              }
              frame condition #1 (active) {
                n88 = case shown="\"Busy\"" w243 {
                  tunnel: w245 -> [w247 w249]
                  tunnel: [w246 w248] -> w244
                  frame "Idle", Default {
                    n89 = call <vilib>:"Unset Busy.vi"("error in (no error)"=w247) -> ("error out"=w246:errorcluster)  [unwired: 10 in]
                  }
                  frame "Busy" {
                    n90 = call <vilib>:"Set Busy.vi"("error in (no error)"=w249) -> ("error out"=w248:errorcluster)  [unwired: 9 in, 1 out]
                  }
                }
              }
            }
            n91 = call <vilib>:"Add State(s) to Queue__jki_lib_state_machine.vi"("State(s) in (\"\")"=w241) -> ("States Out"=w240:string)  [unwired: 14 in]
          }
          frame "UI: Front Panel State" {
            # "Argument"
            # "Set Front Panel Open or Closed\n(Usage: \"UI: Front Panel State >> Open|Close\")"
            n92 = Unbundle By Name(w253) -> ("Core.Current VI Reference"=w252:refnum<vi>)
            n93 = disable-structure shown="Default" {
              disable-tunnel: w255 -> [w261 w284]
              disable-tunnel: [w260 w284] -> w254
              disable-tunnel: w252 -> [w259 _]
              disable-tunnel: w251 -> [w258 _]
              frame condition #0 (active) {
                n94 = case shown="\"Close\"" w258 {
                  tunnel: w261 -> [w265 w278]
                  tunnel: [w267 w279] -> w260
                  tunnel: w259 -> [w266 w276]
                  frame "Open", Default {
                    n95 = property class="VI"(reference=w266, error in=w265) -> (reference out=w263:refnum<vi>, error out=w264:errorcluster, "FP.State"=w262:T5)
                    n96 = case shown="\"Closed\"" w262 {
                      tunnel: [w270 w273] -> w267
                      tunnel: w264 -> [w269 w273]
                      tunnel: w263 -> [w268 _]
                      frame "Closed" {
                        n97 = invoke class="VI" method="FP.Open"(reference=w268, error in=w269, "Activate"=TRUE, "State"=T5."Standard") -> (error out=w270:errorcluster)  [unwired: 1 in, 4 out]
                      }
                      frame Default {
                      }
                    }
                  }
                  frame "Close" {
                    n98 = property class="VI"(reference=w276, error in=w278) -> (reference out=w275:refnum<vi>, error out=w277:errorcluster, "FP.State"=w274:T5)
                    n99 = case shown="Default" w274 {
                      tunnel: [w280 w283] -> w279
                      tunnel: w277 -> [w280 w282]
                      tunnel: w275 -> [_ w281]
                      frame "Invalid", "Closed" {
                      }
                      frame Default {
                        n100 = invoke class="VI" method="FP.Close"(reference=w281, error in=w282) -> (error out=w283:errorcluster)  [unwired: 1 in, 2 out]
                      }
                    }
                  }
                }
              }
              frame condition #1 {
              }
            }
            n101 = call <vilib>:"Add State(s) to Queue__jki_lib_state_machine.vi"("State(s) in (\"\")"=w257) -> ("States Out"=w256:string)  [unwired: 14 in]
          }
          frame "---------- Macro ----------" {
            # "Do not put any code in this frame.\n(It is a separator no-op. You can make a copy of this frame to create a new Macro frame)"
            n102 = call <vilib>:"Add State(s) to Queue__jki_lib_state_machine.vi"("State(s) in (\"\")"=w289) -> ("States Out"=w288:string)  [unwired: 14 in]
          }
          frame "Macro: Initialize" {
            w292 = "UI: Initialize\nMacro: Read UI Config\nAction: Open\n//UI: Front Panel State >> Open"  # UI: Initialize Macro: Read UI Config Action: Open //UI: Front Panel State >> Open
            # "Initialization Macro\n(This is called once, when the VI starts)"
            n103 = call <vilib>:"Add State(s) to Queue__jki_lib_state_machine.vi"("State(s) in Front (\"\")"="Data: Initialize\nInitialize Core Data\nEvents: Register", "State(s) in (\"\")"="Process: Sync", "State(s) at Back (\"\")"=w292) -> ("States Out"=w291:string)  [unwired: 12 in]
            n104 = call <vilib>:"Add State(s) to Queue__jki_lib_state_machine.vi"("State(s) in Front (\"\")"=w291, "State(s) in (\"\")"=w298) -> ("States Out"=w297:string)  [unwired: 13 in]
          }
          frame "Macro: Post Error Handling" {
            # "Clear Last Error?"
            n105 = Unbundle By Name(w300) -> ("Core.Last Error.remaining states"=w302:string, "Core.Shutdown?"=w303:bool)
            n106 = Unbundle By Name(w300) -> ("Core.Last Error.error"=w306:errorcluster)
            n107 = case shown="False" FALSE {
              tunnel: w306 -> [w314 _]
              tunnel: [w314 _] -> w305
              frame False {
              }
              frame True {
              }
            }
            n108 = case shown="True" w303 {
              tunnel: w302 -> [w311 w313]
              tunnel: [w311 w312] -> w299
              frame False {
                # "These are the remaining states (at the moment the error occured). States can be altered according to business logic."
                # "NOT SHUTTING DOWN"
              }
              frame True {
                # "Developer can decide to alter the states but should be aware that during the shutdown process, there are certain states that must be run for the SMO to properly shut itself (and this process) down. As such, one can add states to perform additional clean-ups, but should append the remaining state to be executed."
                # "SHUTTING DOWN"
                n109 = call <vilib>:"Add State(s) to Queue__jki_lib_state_machine.vi"("State(s) in (\"\")"=w313) -> ("States Out"=w312:string)  [unwired: 14 in]
              }
            }
            n110 = Bundle By Name(cluster=w300, "Core.Last Error.error"=w305) -> (w301:T10)
            n111 = call <vilib>:"Add State(s) to Queue__jki_lib_state_machine.vi"("State(s) in Front (\"\")"=w299, "State(s) in (\"\")"=w310) -> ("States Out"=w309:string)  [unwired: 13 in]
          }
          frame "Macro: Read UI Config" {
            # "Do not put any code in this frame.\n(It is a separator no-op. You can make a copy of this frame to create a new Macro frame)"
            n112 = call <vilib>:"Add State(s) to Queue__jki_lib_state_machine.vi"("State(s) in Front (\"\")"="Configuration: Initialize\nConfiguration: Read UI Config File\nUI: Update FP Controls" ("State(s) in Front (\"\")"), "State(s) in (\"\")"=w320) -> ("States Out"=w319:string)  [unwired: 13 in]
          }
          frame "Macro: Write UI Config" {
            # "Do not put any code in this frame.\n(It is a separator no-op. You can make a copy of this frame to create a new Macro frame)"
            n113 = call <vilib>:"Add State(s) to Queue__jki_lib_state_machine.vi"("State(s) in Front (\"\")"="Data: Set UI Cluster\nConfiguration: Write UI Config File" ("State(s) in Front (\"\")"), "State(s) in (\"\")"=w326) -> ("States Out"=w325:string)  [unwired: 13 in]
          }
          frame "Macro: Exit" {
            # "Exit Macro\n(This is called once, when the VI exits)"
            n114 = Unbundle By Name(w328) -> ("Core.Close Panel on Exit?"=w338:bool)
            n115 = Select(t="UI: Front Panel State >> Close", s=w338, f="" ("Empty String Constant")) -> (s? t:f=w335:string)
            n116 = call <vilib>:"Add State(s) to Queue__jki_lib_state_machine.vi"("State(s) in Front (\"\")"="Data: Cleanup\nEvents: Unregister\nProcess: Self Terminate", "State(s) in (\"\")"="Process: Sync", "State(s) at Back (\"\")"="Exit") -> ("States Out"=w330:string)  [unwired: 12 in]
            n117 = call <vilib>:"Add State(s) to Queue__jki_lib_state_machine.vi"("State(s) in Front (\"\")"="Action: Close\nMacro: Write UI Config", "State(s) in (\"\")"=w335, "State(s) at Back (\"\")"=w330) -> ("States Out"=w334:string)  [unwired: 12 in]
            n118 = call <vilib>:"Add State(s) to Queue__jki_lib_state_machine.vi"("State(s) in Front (\"\")"=w334, "State(s) in (\"\")"=w341) -> ("States Out"=w340:string)  [unwired: 13 in]
          }
          frame "---------- Process ----------" {
            # "Template Separator\n(You can make a copy of, or modify, this frame)"
            n119 = call <vilib>:"Add State(s) to Queue__jki_lib_state_machine.vi"("State(s) in (\"\")"=w346) -> ("States Out"=w345:string)  [unwired: 14 in]
          }
          frame "Process: Sync" {
            n120 = Unbundle By Name(w354) -> ("Instrument UI"=w350:refnum<class "Inst UI.Magneto.lvclass">)
            n121 = call <vilib>:"WaitOnProcessSync.vi"("error in (no error)"=w349, "SMO"=w350) -> ("error out"=w348:errorcluster, "Don't run?"=w353:bool)  [unwired: 7 in, 1 out]
            n122 = Select(t="Data: Cleanup\nEvents: Unregister\nExit", s=w353, f="" ("Empty String Constant")) -> (s? t:f=w347:string)
            n123 = call <vilib>:"Add State(s) to Queue__jki_lib_state_machine.vi"("State(s) in Front (\"\")"=w347, "State(s) in (\"\")"=w357) -> ("States Out"=w356:string)  [unwired: 13 in]
          }
          frame "Process: Self Terminate" {
            n124 = Unbundle By Name(w359) -> ("Instrument UI"=w358:refnum<class "Inst UI.Magneto.lvclass">)
            n125 = call <vilib>:"SelfTerminate.vi"("error in (no error)"=w361, "SMO in"=w358) -> ("error out"=w360:errorcluster)  [unwired: 8 in, 1 out]
            n126 = call <vilib>:"Add State(s) to Queue__jki_lib_state_machine.vi"("State(s) in (\"\")"=w364) -> ("States Out"=w363:string)  [unwired: 14 in]
          }
          frame "---------- Events ----------" {
            # "Template Separator\n(You can make a copy of, or modify, this frame)"
            n127 = call <vilib>:"Add State(s) to Queue__jki_lib_state_machine.vi"("State(s) in (\"\")"=w369) -> ("States Out"=w368:string)  [unwired: 14 in]
          }
          frame "Events: Register" {
            # "Expand to add\nmore events"
            # "Base Class Protected Events"
            n128 = Unbundle By Name(w383) -> ("Instrument UI"=w376:refnum<class "Inst UI.Magneto.lvclass">, "Instrument"=w375:refnum<class "Inst.Magneto.lvclass">)
            n129 = call <vilib>:"GetProtectedEvents.vi"("SMO"=w376) -> ("error out"=w379:errorcluster, "SMO Protected Events"=w381:T12)  [unwired: 8 in, 1 out]
            n130 = call <userlib>:"Instrument.GetPublicEvents.vi"("Instrument"=w375) -> ("error out"=w377:errorcluster, "Instrument Public Events"=w378:T13, "Instrument out"=w373:refnum<class "Inst.Magneto.lvclass">)  [unwired: 8 in]
            n131 = call "Inst.Magneto.GetPublicEvents.vi"("Inst.Magneto in"=w373) -> ("error out"=w372:errorcluster, "Inst.Magneto Public Events"=w374:T14)  [unwired: 8 in, 1 out]
            n132 = register-events(w381, w378, w374) -> (reference out=w382:refnum<event-registration>, error out=w371:errorcluster)  [unwired: 2 in]
            n133 = Merge Errors(w371, w372, w377, w379, w370) -> (w380:errorcluster)
            n134 = call <vilib>:"Add State(s) to Queue__jki_lib_state_machine.vi"("State(s) in (\"\")"=w385) -> ("States Out"=w384:string)  [unwired: 14 in]
          }
          frame "Events: Unregister" {
            n135 = Unregister For Events(event registration refnum=w388, error in=w387) -> (error out=w386:errorcluster)
            n136 = call <vilib>:"Add State(s) to Queue__jki_lib_state_machine.vi"("State(s) in (\"\")"=w391) -> ("States Out"=w390:string)  [unwired: 14 in]
          }
          frame "---------- Configuration ----------" {
            # "Do not put any code in this frame.\n(It is a separator no-op. You can make a copy of this frame to create a new UI frame)"
            n137 = call <vilib>:"Add State(s) to Queue__jki_lib_state_machine.vi"("State(s) in (\"\")"=w396) -> ("States Out"=w395:string)  [unwired: 14 in]
          }
          frame "Configuration: Initialize" {
            # "Do not put any code in this frame.\n(It is a separator no-op. You can make a copy of this frame to create a new UI frame)"
            n138 = Unbundle By Name(w404) -> ("Configuration"=w402:refnum<class "Configuration.lvclass">, "Instrument"=w403:refnum<class "Inst.Magneto.lvclass">)
            n139 = call <vilib>:"GetName.vi"("error in (no error)"=w406, "SMO"=w403) -> ("error out"=w405:errorcluster, "Name"=w407:string)  [unwired: 6 in, 2 out]
            n140 = call <userlib>:"Default Path.vi"("error in (no error)"=w405, "Folder Name [Application Name]"=w407, "Configuration in"=w402) -> ("error out"=w398:errorcluster, "Configuration out"=w401:refnum<class "Configuration.lvclass">)  [unwired: 7 in]
            n141 = call <userlib>:"Write Section.vi"("error in (no error)"=w398, "Section"="UI", "Configuration in"=w401) -> ("error out"=w397:errorcluster, "Configuration out"=w400:refnum<class "Configuration.lvclass">)  [unwired: 7 in]
            n142 = Bundle By Name(cluster=w404, "Configuration"=w400) -> (w408:T10)
            n143 = call <vilib>:"Add State(s) to Queue__jki_lib_state_machine.vi"("State(s) in (\"\")"=w411) -> ("States Out"=w410:string)  [unwired: 14 in]
          }
          frame "Configuration: Write UI Config File" {
            # "Do not put any code in this frame.\n(It is a separator no-op. You can make a copy of this frame to create a new Data frame)"
            n144 = Unbundle By Name(w416) -> ("Configuration"=w413:refnum<class "Configuration.lvclass">, "UI Cluster"=w415:T8)
            n145 = call <userlib>:"Write Configuration.vi"("error in (no error)"=w412, "Variant"=w415, "Configuration in"=w413) -> ("error out"=w414:errorcluster)  [unwired: 7 in, 1 out]
            n146 = call <vilib>:"Add State(s) to Queue__jki_lib_state_machine.vi"("State(s) in (\"\")"=w419) -> ("States Out"=w418:string)  [unwired: 14 in]
          }
          frame "Configuration: Read UI Config File" {
            # "Do not put any code in this frame.\n(It is a separator no-op. You can make a copy of this frame to create a new UI frame)"
            n147 = Unbundle By Name(w422) -> ("UI Cluster"=w425:T8, "Configuration"=w428:refnum<class "Configuration.lvclass">)
            n148 = call <userlib>:"Read Configuration.vi"("INI Fomatted Cluster Type"=w425, "error in (no error)"=w424, "Configuration in"=w428) -> ("error out"=w427:errorcluster, "Configuration"=w426:variant)  [unwired: 6 in, 1 out]
            n149 = Variant To Data(error in=w427, type=w425, Variant=w426) -> (data=w421:T8, error out=w423:errorcluster)
            n150 = Bundle By Name(cluster=w422, "UI Cluster"=w421) -> (w420:T10)
            n151 = call <vilib>:"Add State(s) to Queue__jki_lib_state_machine.vi"("State(s) in (\"\")"=w431) -> ("States Out"=w430:string)  [unwired: 14 in]
          }
          frame "---------- Action ----------" {
            n152 = Unbundle By Name(w433) -> ("Instrument"=w434:refnum<class "Inst.Magneto.lvclass">)
            n153 = Bundle By Name(cluster=w433, "Instrument"=w434) -> (w432:T10)
            n154 = call <vilib>:"Add State(s) to Queue__jki_lib_state_machine.vi"("State(s) in (\"\")"=w438) -> ("States Out"=w437:string)  [unwired: 14 in]
          }
          frame "Action: Notify UI Closed" {
            # "Notify that the UI has been closed"
            n155 = Unbundle By Name(w439) -> ("Instrument UI"=w442:refnum<class "Inst UI.Magneto.lvclass">)
            n156 = call <vilib>:"Hide.vi"("error in (no error)"=w441, "SMO.UI"=w442) -> ("error out"=w440:errorcluster)  [unwired: 8 in, 1 out]
            n157 = call <vilib>:"Add State(s) to Queue__jki_lib_state_machine.vi"("State(s) in (\"\")"=w445) -> ("States Out"=w444:string)  [unwired: 14 in]
          }
          frame "Action: getAll" {
            n158 = Unbundle By Name(w449) -> ("getAll"=w447:T3, "Instrument"=w452:refnum<class "Inst.Magneto.lvclass">)
            n159 = call "GET ALL.vim"("type"=w447, "error in (no error)"=w450, "Instrument in"=w452) -> ("error out"=w454:errorcluster, "getAll"=w446:T3, "Instrument out"=w448:refnum<class "Inst.Magneto.lvclass">)  [unwired: 6 in]
            "error out 2" <- w454
            n160 = Bundle By Name(cluster=w449, "Instrument"=w448, "getAll"=w446) -> (w451:T10)
            n161 = call <vilib>:"Add State(s) to Queue__jki_lib_state_machine.vi"("State(s) in Front (\"\")"="" ("State(s) in Front (\"\")"), "State(s) in (\"\")"=w457) -> ("States Out"=w456:string)  [unwired: 13 in]
          }
          frame "Action: Open" {
            n162 = Unbundle By Name(w464) -> ("Instrument"=w462:refnum<class "Inst.Magneto.lvclass">)
            n163 = call <userlib>:"Write Client Type.vi"("error in (no error)"=w459, "Client Type"=Client_Type--Enum."Local", "Instrument in"=w462) -> ("error out"=w460:errorcluster, "Instrument out"=w461:refnum<class "Inst.Magneto.lvclass">)  [unwired: 7 in]
            n164 = call-dynamic "Open.vi"("error in (no error)"=w460, "Inst.Magneto in"=w461) -> ("error out"=w467:errorcluster, "Inst.Magneto out"=w463:refnum<class "Inst.Magneto.lvclass">)  [unwired: 8 in]
            n165 = Bundle By Name(cluster=w464, "Instrument"=w463) -> (w465:T10)
            n166 = call <vilib>:"Add State(s) to Queue__jki_lib_state_machine.vi"("State(s) in Front (\"\")"="" ("State(s) in Front (\"\")"), "State(s) in (\"\")"=w470) -> ("States Out"=w469:string)  [unwired: 13 in]
          }
          frame "Action: Close" {
            n167 = Unbundle By Name(w472) -> ("Instrument"=w475:refnum<class "Inst.Magneto.lvclass">)
            n168 = call-dynamic "Close.vi"("error in (no error)"=w473, "Inst.Magneto in"=w475) -> ("error out"=w477:errorcluster, "Inst.Magneto out"=w471:refnum<class "Inst.Magneto.lvclass">)  [unwired: 8 in]
            n169 = Bundle By Name(cluster=w472, "Instrument"=w471) -> (w474:T10)
            n170 = call <vilib>:"Add State(s) to Queue__jki_lib_state_machine.vi"("State(s) in Front (\"\")"="" ("State(s) in Front (\"\")"), "State(s) in (\"\")"=w480) -> ("States Out"=w479:string)  [unwired: 13 in]
          }
          frame "Action: Send Message to Instrument" {
            # "Send a message (command, data, etc) to the Instrument:process.vi"
            n171 = Unbundle By Name(w486) -> ("Instrument"=w485:refnum<class "Inst.Magneto.lvclass">, "Message.Command"=w481:string)
            n172 = call <userlib>:"Instrument.MessageToProcess.vi"("error in (no error)"=w483, "Command"=w481, "Instrument"=w485) -> ("error out"=w482:errorcluster, "Instrument out"=w484:refnum<class "Inst.Magneto.lvclass">)  [unwired: 7 in]
            n173 = Bundle By Name(cluster=w486, "Instrument"=w484) -> (w487:T10)
            n174 = call <vilib>:"Add State(s) to Queue__jki_lib_state_machine.vi"("State(s) in Front (\"\")"="" ("State(s) in Front (\"\")"), "State(s) in (\"\")"=w491) -> ("States Out"=w490:string)  [unwired: 13 in]
          }
          frame "Action: GetRead" {
            # "Send a message (command, data, etc) to the Instrument:process.vi"
            n175 = Unbundle By Name(w497) -> ("Instrument"=w496:refnum<class "Inst.Magneto.lvclass">)
            n176 = call <userlib>:"Instrument.MessageToProcess.vi"("error in (no error)"=w494, "Command"="GetRead", "Instrument"=w496) -> ("error out"=w493:errorcluster, "Instrument out"=w495:refnum<class "Inst.Magneto.lvclass">)  [unwired: 7 in]
            n177 = Bundle By Name(cluster=w497, "Instrument"=w495) -> (w498:T10)
            n178 = call <vilib>:"Add State(s) to Queue__jki_lib_state_machine.vi"("State(s) in Front (\"\")"="" ("State(s) in Front (\"\")"), "State(s) in (\"\")"=w502) -> ("States Out"=w501:string)  [unwired: 13 in]
          }
          frame "Action: Send Message to Child" {
            # "Send a message (command, data, etc) to the Instrument.Child:process.vi"
            n179 = Unbundle By Name(w507) -> ("Instrument"=w506:refnum<class "Inst.Magneto.lvclass">)  [unwired: 1 out]
            n180 = call "Inst.Magneto.MessageToProcess.vi"("error in (no error)"=w504, "Inst.Magneto in"=w506) -> ("error out"=w503:errorcluster, "Inst.Magneto out"=w505:refnum<class "Inst.Magneto.lvclass">)  [unwired: 8 in]
            n181 = Bundle By Name(cluster=w507, "Instrument"=w505) -> (w508:T10)
            n182 = call <vilib>:"Add State(s) to Queue__jki_lib_state_machine.vi"("State(s) in Front (\"\")"="" ("State(s) in Front (\"\")"), "State(s) in (\"\")"=w512) -> ("States Out"=w511:string)  [unwired: 13 in]
          }
        }
      }
    }
    frame Error {
    }
  }
  n183 = call-parent "Process.vi"("error in"=w5, "Instrument UI in"=w4) -> ("error out"=w2:errorcluster, "Instrument UI out"=→"Inst UI.Magneto out":refnum<class "Inst UI.Magneto.lvclass">)  [unwired: 8 in]
  n184 = Merge Errors(w2, w1) -> (→"error out":errorcluster)
